vi "Configure Parameter.vi"(8 "error in (no error)":errorcluster, 10 "Configure Parameter":T1={"Temp Parameter"={"Temperature setpoint"=40.0, "upper limit"=80.0, "lower limit"=0.0}, "Humidity Parameter"={"Humidity setpoint"=50.0, "upper limit"=80.0, "lower limit"=0.0}}, 11 "Abstract in":refnum<class "Abstract.lvclass">) -> (0 "error out":errorcluster, 3 "Abstract out":refnum<class "Abstract.lvclass">)   [LabVIEW 2021, in "Environment Chamber.lvlib" / "Abstract.lvclass"]
uses:
  Abstract.lvclass
  Configure Parameter.ctl
  Environment Chamber.lvlib
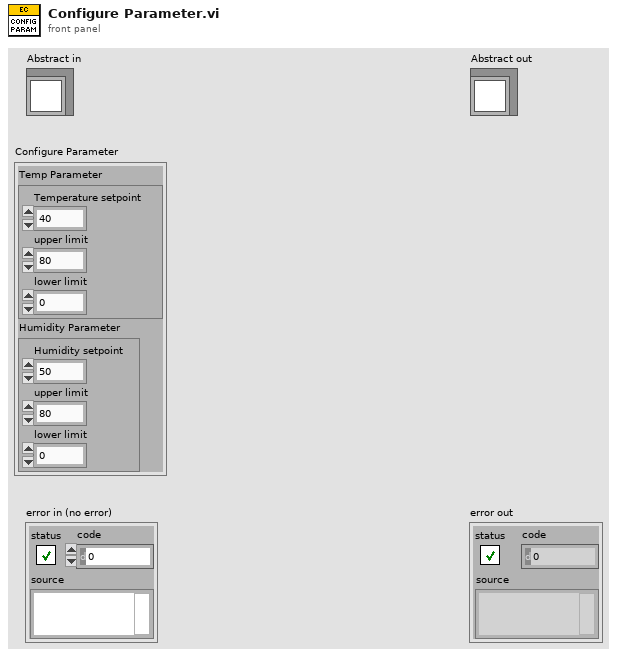
[diagram p1: front panel]
types:
  T1 = typedef "Environment Chamber.lvlib/Configure Parameter.ctl" = cluster{"Temp Parameter":cluster{"Temperature setpoint":dbl, "upper limit":dbl, "lower limit":dbl}, "Humidity Parameter":cluster{"Humidity setpoint":dbl, "upper limit":dbl, "lower limit":dbl}}
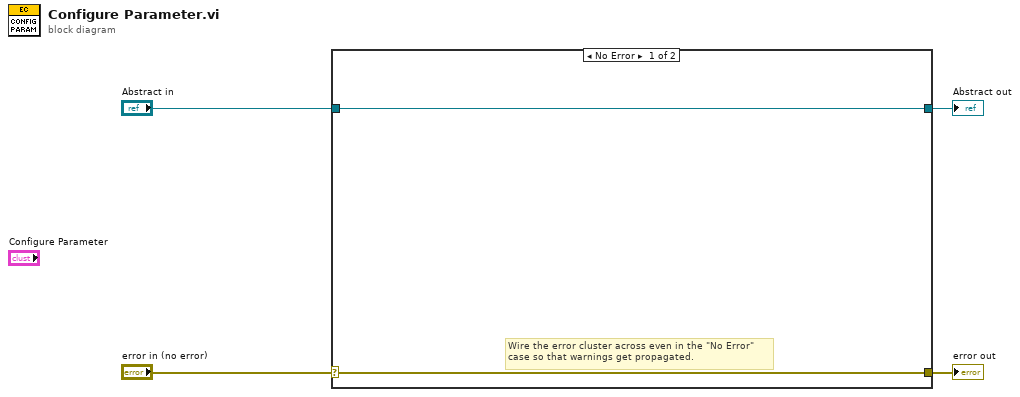
[diagram p0: block diagram]
diagram:
  n1 = case shown="No Error" "error in (no error)" {
    selector: "error in (no error)" -> [w5 w8]
    tunnel: [w5 w8] -> w3
    tunnel: [w6 w7] -> w1
    tunnel: "Abstract in" -> [w6 w7]
    frame No Error {
      # "Wire the error cluster across even in the \"No Error\"\ncase so that warnings get propagated."
    }
    frame Error {
    }
  }
  "error out" <- w3
  "Abstract out" <- w1
